vi "NI 9211_TASK_TC.vi"(8 "error in":errorcluster, 11 "MODULE NAME":string="cDAQ_NICOTRAMod4") -> (0 "error out":errorcluster, 3 "task out":refnum<k21>)   [LabVIEW 2019]
uses:
  <vilib>/DAQmx/create/channels.llb/DAQmx Create Channel (TEDS-AI-Temperature-Thermocouple).vi
  <vilib>/DAQmx/create/channels.llb/DAQmx Create Channel (AI-Temperature-Thermocouple).vi
  <vilib>/DAQmx/configure/timing.llb/DAQmx Timing (Sample Clock).vi
  <resource>/objmgr/daqmx.rc
  <vilib>/DAQmx/create/channels.llb/DAQmx Create Channel (AI-Temperature-RTD).vi
panel:
  out "Numeric 2":i32
  out "Numeric":i32
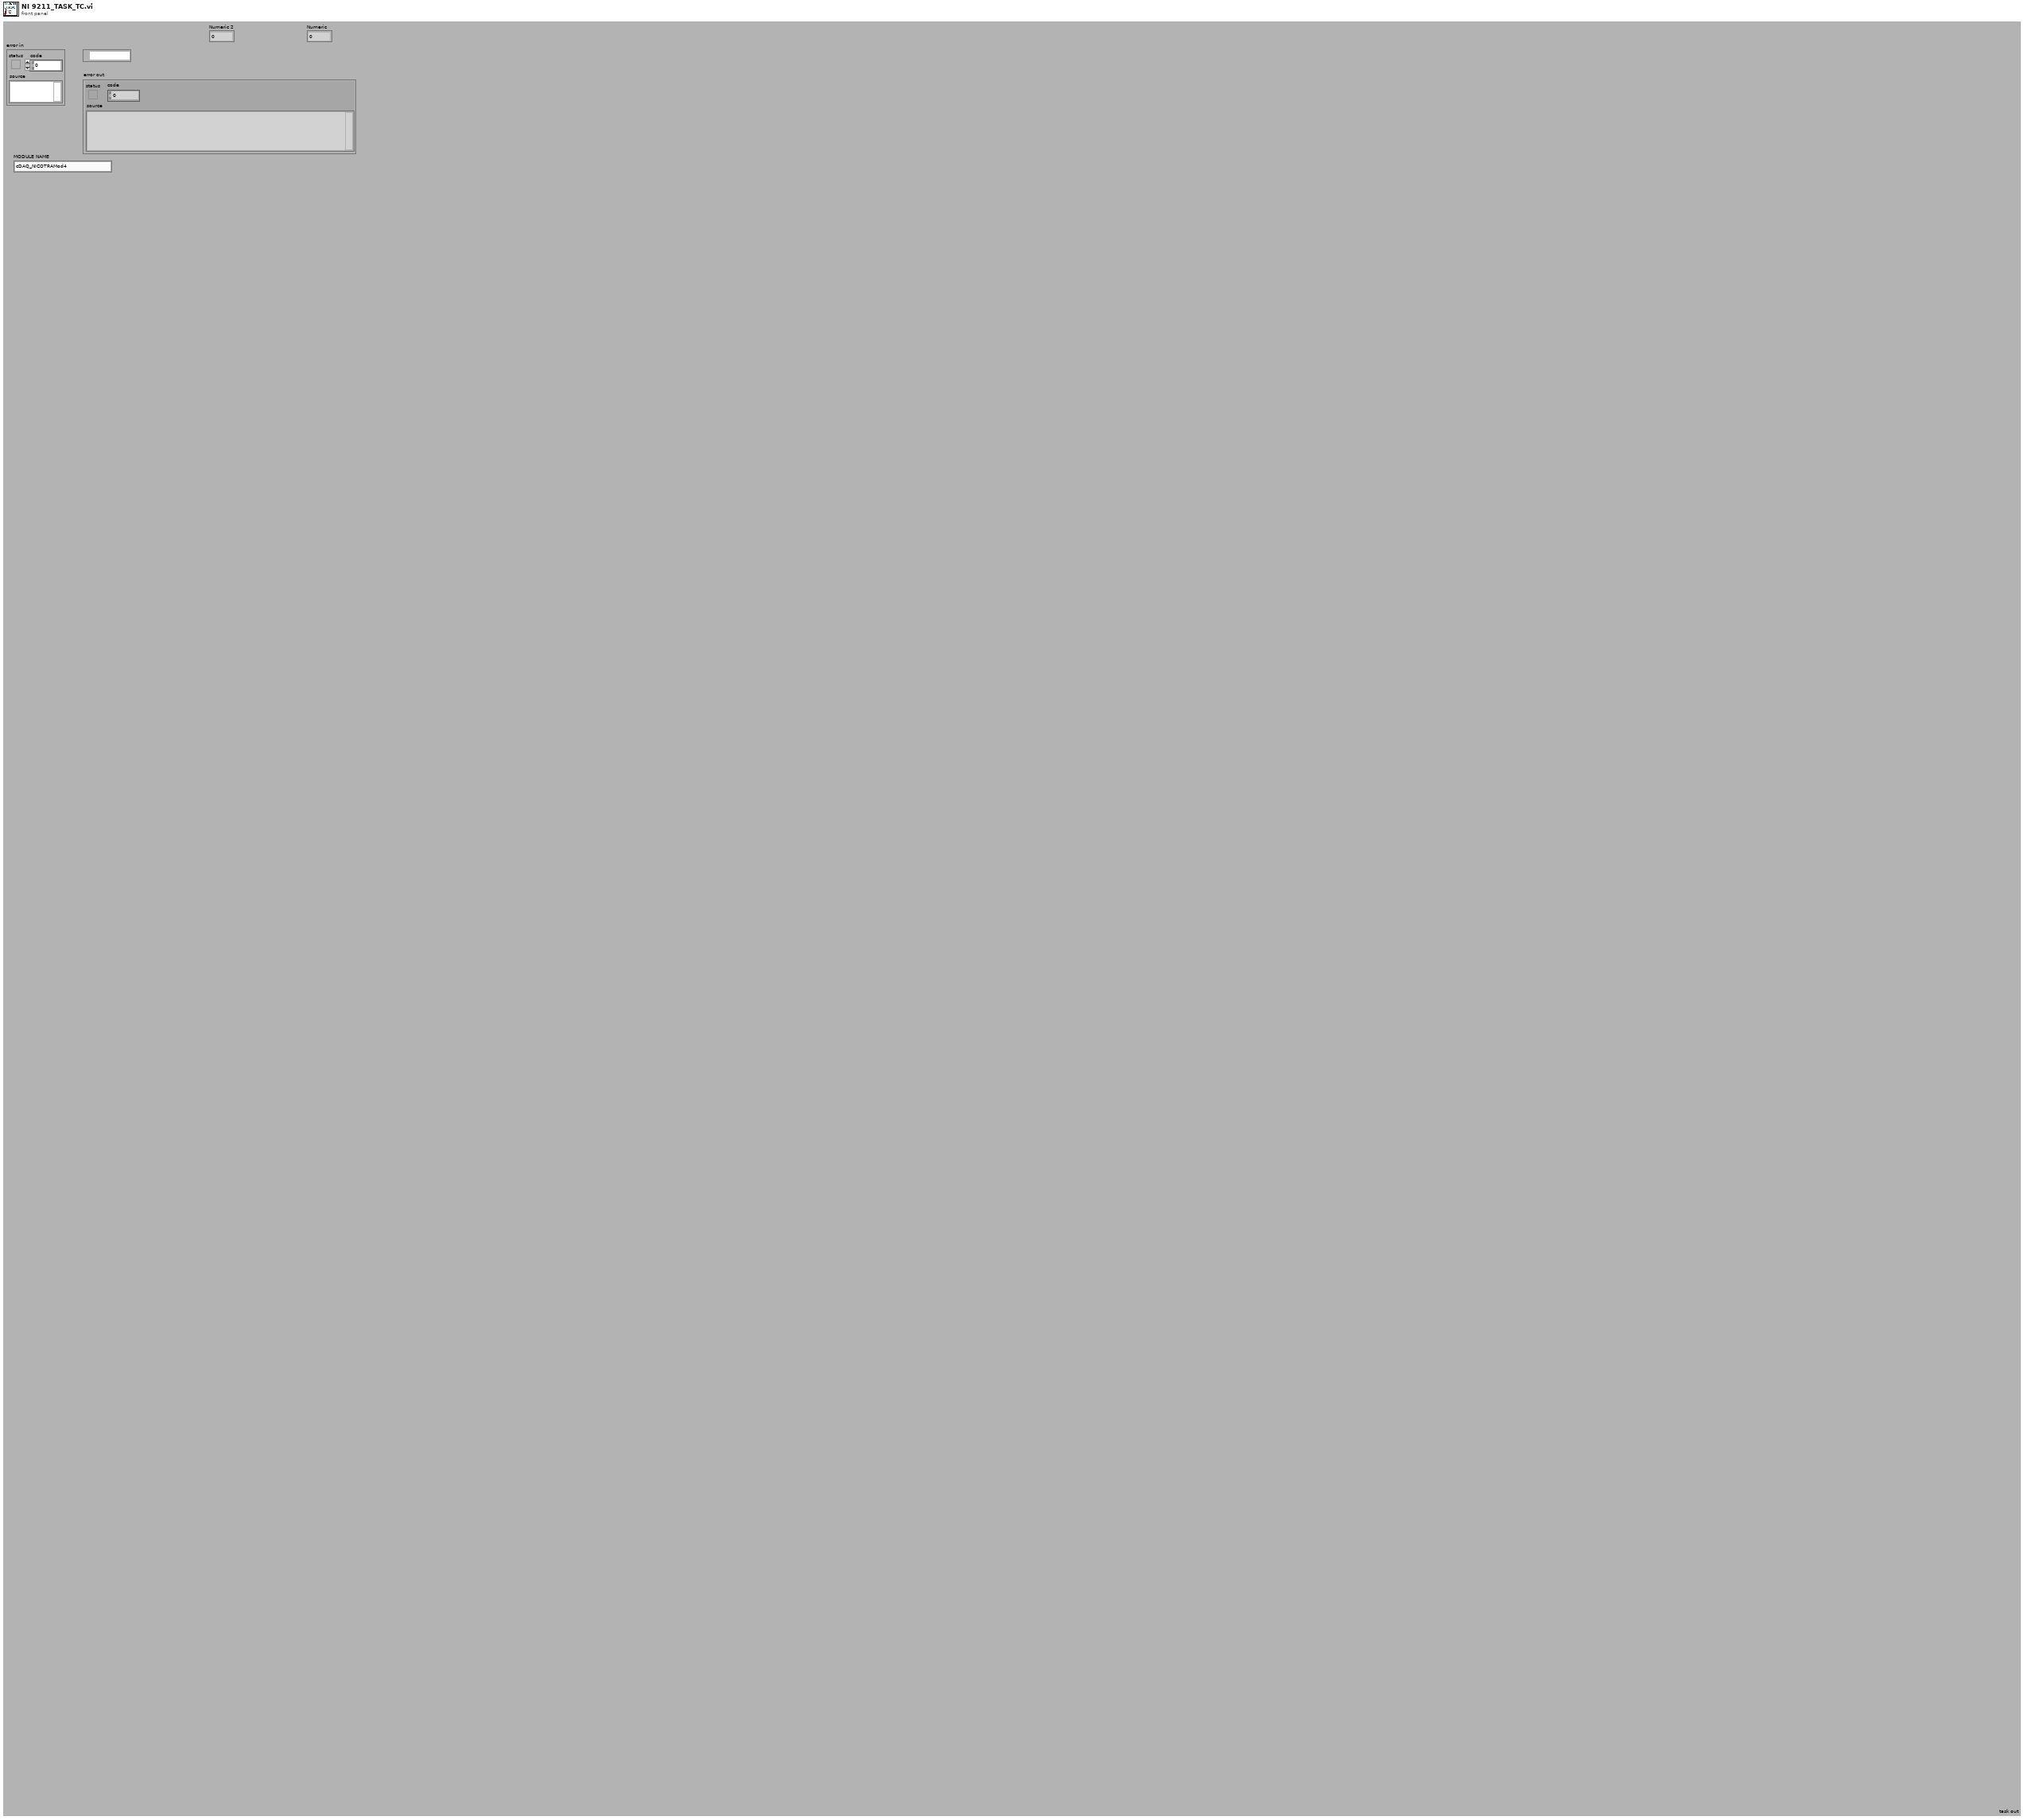
[diagram p1: front panel]
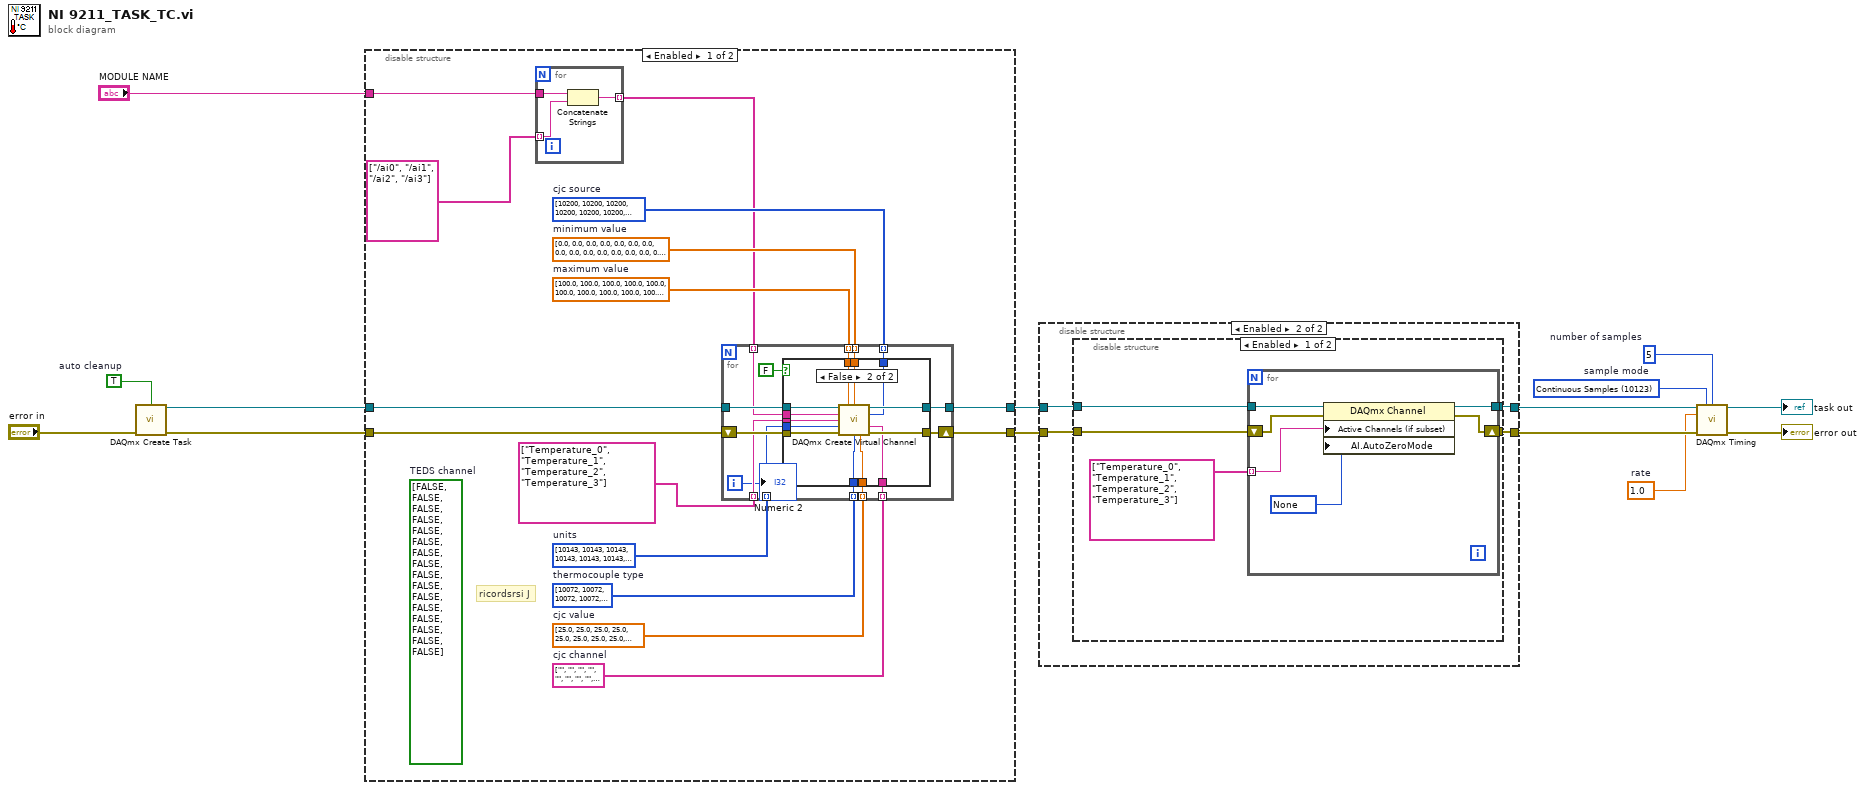
[diagram p0: block diagram]
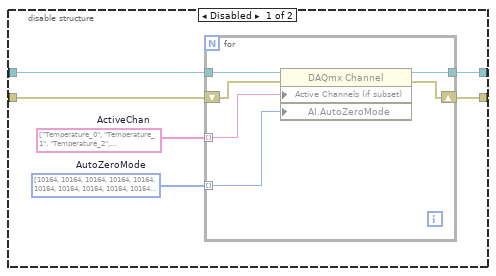
[diagram p2: hidden frame]
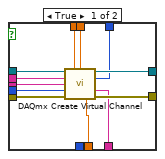
[diagram p4: hidden frame]
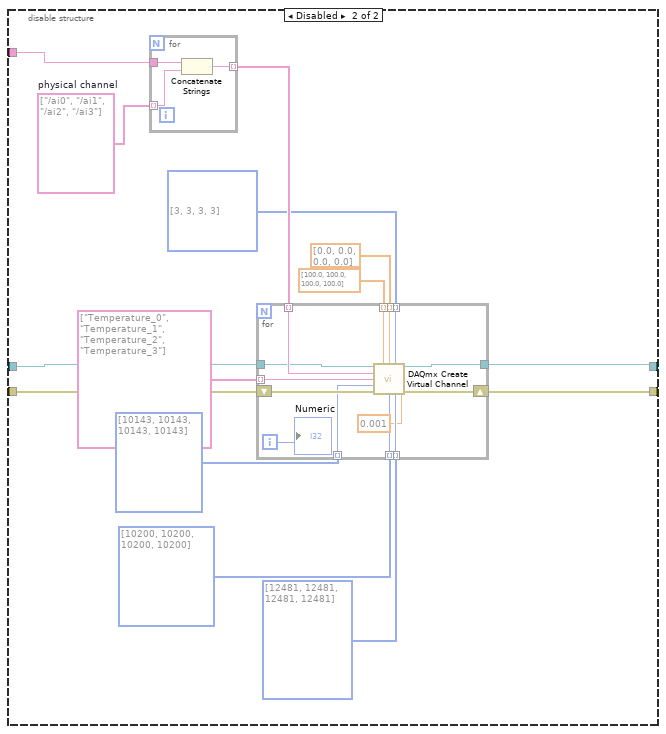
[diagram p5: hidden frame]
diagram:
  w5 = 10123 items=["Finite Samples"=10178, "Continuous Samples"=10123, "Hardware Timed Single Point"=12522]  # sample mode
  w6 = 5  # number of samples
  w7 = 1.0  # rate
  w13 = TRUE  # auto cleanup
  n1 = call <vilib>:"DAQmx Create Task.vi"("auto cleanup"=w13, "error in"="error in") -> ("task out"=w12:refnum<k21>, "error out"=w14:errorcluster)  [unwired: 12 in]
  n2 = disable-structure shown="Enabled" {
    disable-tunnel: w14 -> [w29 w76]
    disable-tunnel: w12 -> [w28 w83]
    disable-tunnel: [w23 w77] -> w11
    disable-tunnel: [w19 w78] -> w9
    disable-tunnel: "MODULE NAME" -> [w18 w85]
    frame Enabled {
      (unwired) bool[] [FALSE, FALSE, FALSE, FALSE, FALSE, FALSE, FALSE, FALSE, FALSE, FALSE, FALSE, FALSE, FALSE, FALSE, FALSE, FALSE]  # TEDS channel
      w21 = dbl[] [25.0, 25.0, 25.0, 25.0, 25.0, 25.0, 25.0, 25.0, 25.0, 25.0, 25.0, 25.0, 25.0, 25.0, 25.0, 25.0]  # cjc value
      w20 = string[] ["", "", "", "", "", "", "", "", "", "", "", "", "", "", "", ""]  # cjc channel
      w25 = i32[] [10072, 10072, 10072, 10072, 10072, 10072, 10072, 10072, 10073, 10073, 10073, 10073, 10073, 10073, 10073, 10072] items=["J"=10072, "K"=10073, "N"=10077, "R"=10082, "S"=10085, "T"=10086, "B"=10047, "E"=10055]  # thermocouple type
      w24 = i32[] [10143, 10143, 10143, 10143, 10143, 10143, 10143, 10143, 10143, 10143, 10143, 10143, 10143, 10143, 10143, 10143] items=["deg C"=10143, "deg F"=10144, "Kelvins"=10325, "deg R"=10145, "From Custom Scale"=10065]  # units
      w26 = dbl[] [100.0, 100.0, 100.0, 100.0, 100.0, 100.0, 100.0, 100.0, 100.0, 100.0, 100.0, 100.0, 100.0, 100.0, 100.0, 100.0]  # maximum value
      w27 = dbl[] [0.0, 0.0, 0.0, 0.0, 0.0, 0.0, 0.0, 0.0, 0.0, 0.0, 0.0, 0.0, 0.0, 0.0, 0.0, 0.0]  # minimum value
      w22 = u32[] [10200, 10200, 10200, 10200, 10200, 10200, 10200, 10200, 10200, 10200, 10200, 10200, 10200, 10200, 10200, 10200] items=["Internal"=10200, "Constant Value"=10116, "Channel"=10113]  # cjc source
      # "ricordsrsi J"
      n3 = for {
        tunnel: string[] ["/ai0", "/ai1", "/ai2", "/ai3"] -> [w31] mode=indexing
        tunnel: w18 -> [w32]
        tunnel: [w30] -> w17 mode=indexing
        n4 = Concatenate Strings(w32, w31) -> (w30:string)
      }
      n5 = for {
        tunnel: w28 -> [w45]
        tunnel: w27 -> [w46] mode=indexing
        tunnel: w26 -> [w47] mode=indexing
        tunnel: w25 -> [w35] mode=indexing
        tunnel: w24 -> [w39] mode=indexing
        tunnel: string[] ["Temperature_0", "Temperature_1", "Temperature_2", "Temperature_3"] -> [w41] mode=indexing
        tunnel: w17 -> [w40] mode=indexing
        tunnel: [w43] -> w19
        tunnel: w22 -> [w38] mode=indexing
        tunnel: w21 -> [w37] mode=indexing
        tunnel: w20 -> [w36] mode=indexing
        shift-right: [w42] -> w23
        shift-left: w29 -> [w44]
        i -> [w33]
        n6 = case shown="False" FALSE {
          tunnel: w47 -> [w59 w72]
          tunnel: w46 -> [w58 w71]
          tunnel: w45 -> [w57 w70]
          tunnel: w44 -> [w56 w69]
          tunnel: [w55 w68] -> w43
          tunnel: [w54 w67] -> w42
          tunnel: w41 -> [w53 w66]
          tunnel: w40 -> [w52 w65]
          tunnel: w39 -> [w51 w64]
          tunnel: w38 -> [w50 w63]
          tunnel: w37 -> [w49 w62]
          tunnel: w36 -> [w48 w61]
          tunnel: w35 -> [_ w60]
          frame True {
            n7 = call-poly <vilib>:"DAQmx Create Virtual Channel.vi"("task in"=w57, "maximum value"=w59, "minimum value"=w58, "physical channels"=w52, "cjc source"=w50, "name to assign"=w53, "units"=w51, "cjc channel"=w48, "error in"=w56, "cjc value"=w49) -> ("task out"=w55:refnum<k21>, "error out"=w54:errorcluster)  [unwired: 4 in]
          }
          frame False {
            n8 = call-poly <vilib>:"DAQmx Create Virtual Channel.vi"("task in"=w70, "maximum value"=w72, "minimum value"=w71, "physical channels"=w65, "cjc source"=w63, "name to assign"=w66, "units"=w64, "cjc channel"=w61, "error in"=w69, "thermocouple type"=w60, "cjc value"=w62) -> ("task out"=w68:refnum<k21>, "error out"=w67:errorcluster)  [unwired: 3 in]
          }
        }
        "Numeric 2" <- w33
      }
    }
    frame Disabled {
      w74 = i32[] [12481, 12481, 12481, 12481] items=["Pt3750"=12481, "Pt3851"=10071, "Pt3911"=12482, "Pt3916"=10069, "Pt3920"=10053, "Pt3928"=12483, "Custom"=10137]
      w73 = i32[] [10200, 10200, 10200, 10200] items=["Internal"=10200, "External"=10167, "None"=10230]
      w75 = i32[] [10143, 10143, 10143, 10143] items=["Deg C"=10143, "Deg F"=10144, "Kelvins"=10325, "Deg R"=10145, "From Custom Scale"=10065]
      w81 = i32[] [3, 3, 3, 3] items=["2-Wire"=2, "3-Wire"=3, "4-Wire"=4]
      w86 = string[] ["/ai0", "/ai1", "/ai2", "/ai3"]  # physical channel
      n9 = for {
        tunnel: w86 -> [w102] mode=indexing
        tunnel: w85 -> [w103]
        tunnel: [w101] -> w84 mode=indexing
        n10 = Concatenate Strings(w103, w102) -> (w101:string)
      }
      n11 = for {
        tunnel: [w99] -> w78
        shift-right: [w98] -> w77
        shift-left: w76 -> [w100]
        tunnel: w84 -> [w97] mode=indexing
        tunnel: w83 -> [w96]
        tunnel: string[] ["Temperature_0", "Temperature_1", "Temperature_2", "Temperature_3"] -> [w95] mode=indexing
        tunnel: w81 -> [w94] mode=indexing
        tunnel: dbl[] [0.0, 0.0, 0.0, 0.0] -> [w93] mode=indexing
        tunnel: dbl[] [100.0, 100.0, 100.0, 100.0] -> [w92] mode=indexing
        tunnel: w75 -> [w91] mode=indexing
        tunnel: w74 -> [w90] mode=indexing
        tunnel: w73 -> [w89] mode=indexing
        i -> [w88]
        n12 = call-poly <vilib>:"DAQmx Create Virtual Channel.vi"("task in"=w96, "maximum value"=w92, "minimum value"=w93, "resistance configuration"=w94, "physical channels"=w97, "name to assign"=w95, "units"=w91, "current excitation value"=0.001, "error in"=w100, "current excitation source"=w89, "rtd type"=w90) -> ("task out"=w99:refnum<k21>, "error out"=w98:errorcluster)  [unwired: 3 in]
        "Numeric" <- w88
      }
    }
  }
  n13 = disable-structure shown="Enabled" {
    disable-tunnel: w11 -> [w109 w119]
    disable-tunnel: [w107 w116] -> w10
    disable-tunnel: w9 -> [w105 w118]
    disable-tunnel: [w104 w117] -> w8
    frame Disabled {
      w106 = i32[] [10164, 10164, 10164, 10164, 10164, 10164, 10164, 10164, 10164, 10164, 10164, 10164, 10164, 10164, 10164, 10164] items=["None"=10230, "Once"=10244, "Every Sample"=10164]  # AutoZeroMode
      w108 = string[] ["Temperature_0", "Temperature_1", "Temperature_2", "Temperature_3", "Temperature_4", "Temperature_5", "Temperature_6", "Temperature_7", "Temperature_8", "Temperature_9", "Temperature_10", "Temperature_11", "Temperature_12", "Temperature_13", "Temperature_14", "Temperature_15"]  # ActiveChan
      n14 = for {
        tunnel: w105 -> [w113]
        tunnel: w108 -> [w114] mode=indexing
        shift-right: [w115] -> w107
        shift-left: w109 -> [w110]
        tunnel: [w112] -> w104
        tunnel: w106 -> [w111] mode=indexing
        n15 = property class="DAQmx Channel"(reference=w113, error in=w110, "Active Channels (if subset)"=w114, "AI.AutoZeroMode"=w111) -> (reference out=w112:refnum<k21>, error out=w115:errorcluster)
      }
    }
    frame Enabled {
      n16 = disable-structure shown="Enabled" {
        disable-tunnel: w119 -> [w124 w131]
        disable-tunnel: w118 -> [w123 w132]
        disable-tunnel: [w122 w132] -> w117
        disable-tunnel: [w121 w131] -> w116
        frame Enabled {
          n17 = for {
            tunnel: w123 -> [w128]
            tunnel: string[] ["Temperature_0", "Temperature_1", "Temperature_2", "Temperature_3"] -> [w129] mode=indexing
            shift-right: [w130] -> w121
            shift-left: w124 -> [w126]
            tunnel: [w127] -> w122
            w125 = 10230 items=["None"=10230, "Once"=10244, "Every Sample"=10164] ("AI.AutoZeroMode")
            n18 = property class="DAQmx Channel"(reference=w128, error in=w126, "Active Channels (if subset)"=w129, "AI.AutoZeroMode"=w125) -> (reference out=w127:refnum<k21>, error out=w130:errorcluster)
          }
        }
        frame Disabled {
        }
      }
    }
  }
  n19 = call-poly <vilib>:"DAQmx Timing.vi"("task/channels in"=w8, "sample mode"=w5, "samples per channel"=w6, "rate"=w7, "error in"=w10) -> ("task out"=→"task out":refnum<k21>, "error out"=→"error out":errorcluster)  [unwired: 9 in]
